vi "Parse Response.vi"(6 "Command String (Hex)":string, 8 "error in (no error)":errorcluster, 10 "Response String (Hex)":string, 11 "Hitronics in":refnum<class "Hitronics.lvclass">) -> (0 "error out":errorcluster, 2 "Response":string, 3 "Hitronics out":refnum<class "Hitronics.lvclass">)   [LabVIEW 2018, in "Hitronics.lvlib" / "Hitronics.lvclass"]
uses:
  Hitronics.lvclass
  Hitronics.lvclass/Hitronics.ctl
panel:
  out "Data":string
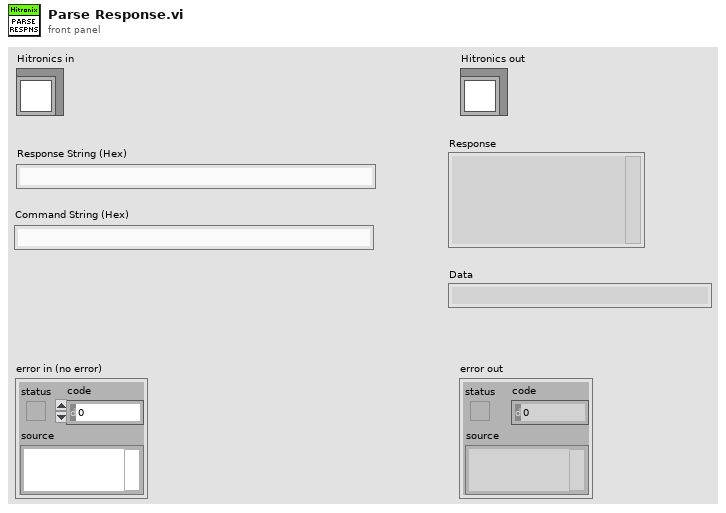
[diagram p1: front panel]
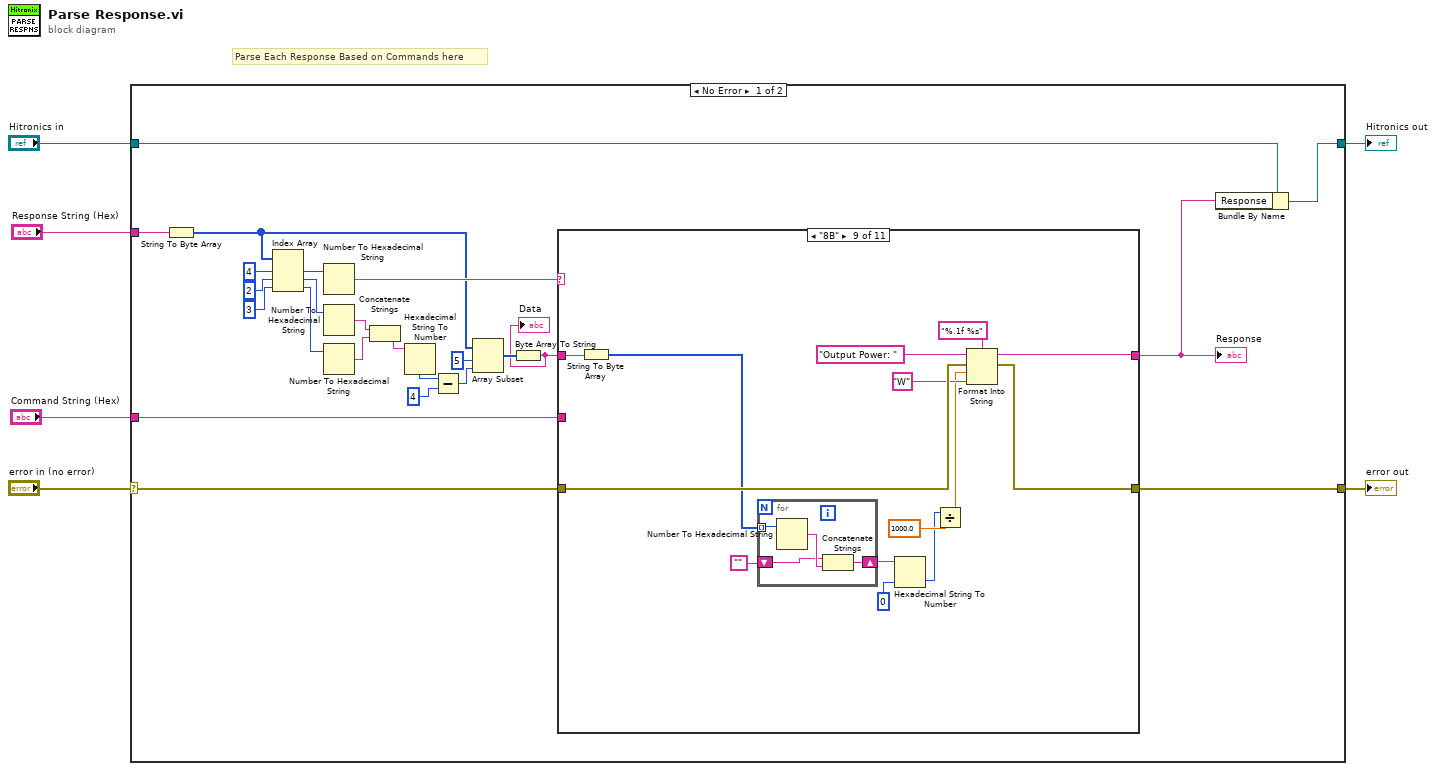
[diagram p0: block diagram]
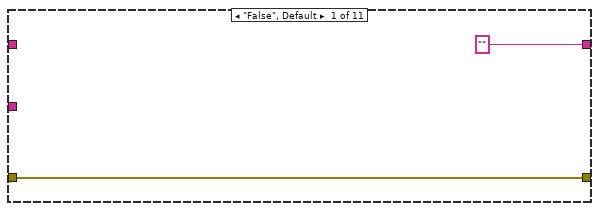
[diagram p2: hidden frame]
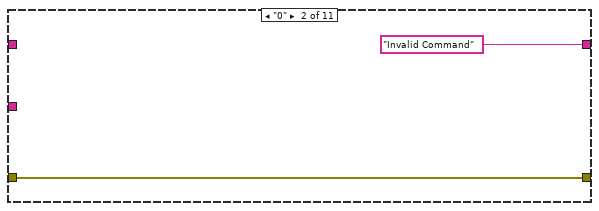
[diagram p3: hidden frame]
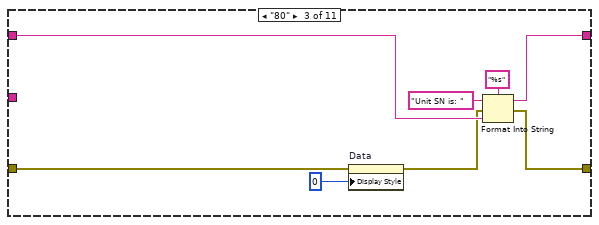
[diagram p4: hidden frame]
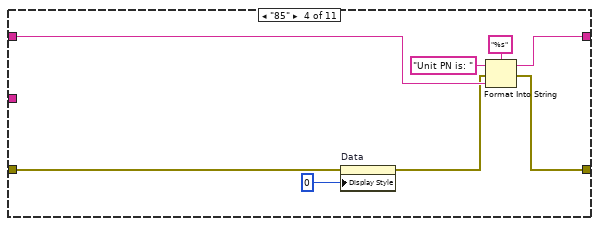
[diagram p5: hidden frame]
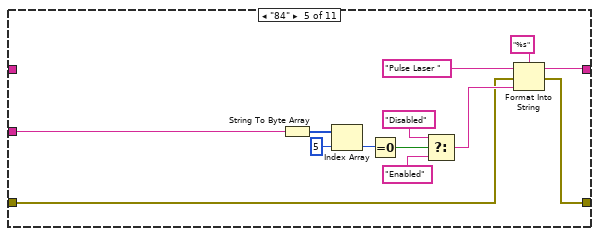
[diagram p6: hidden frame]
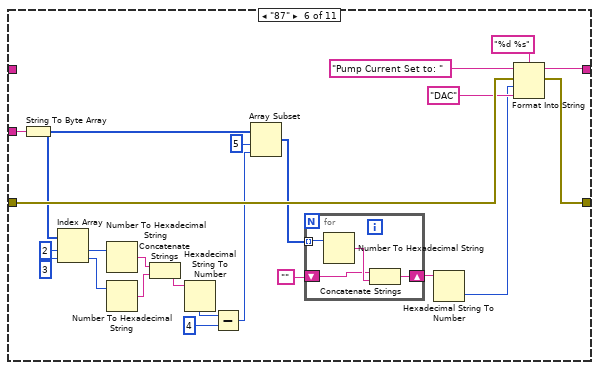
[diagram p7: hidden frame]
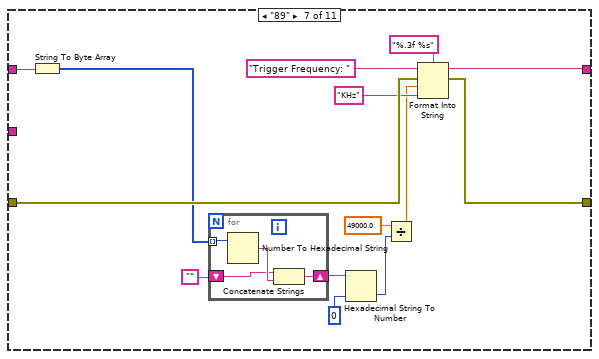
[diagram p8: hidden frame]
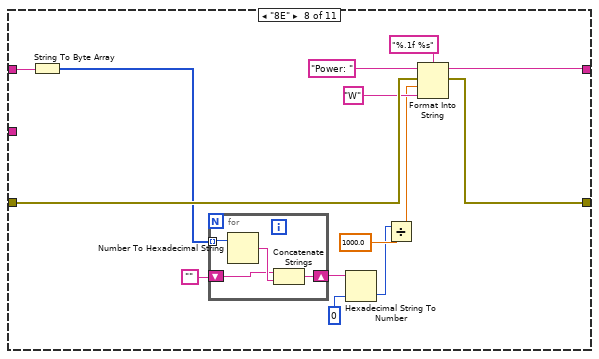
[diagram p9: hidden frame]
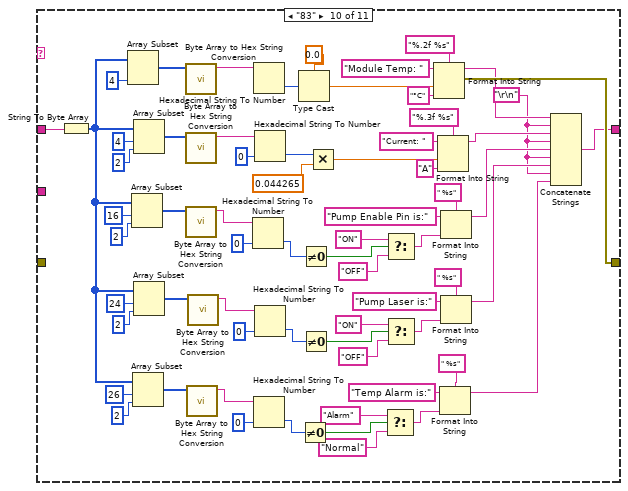
[diagram p10: hidden frame]
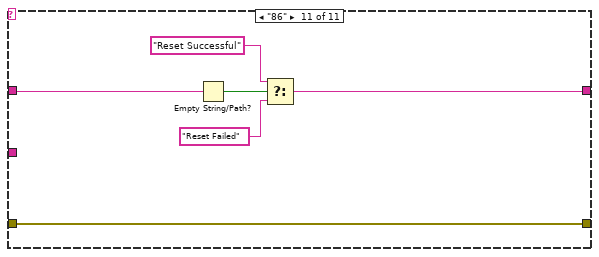
[diagram p11: hidden frame]
diagram:
  # "Parse Each Response Based on Commands here"
  n1 = case shown="No Error" "error in (no error)" {
    selector: "error in (no error)" -> [w12 w218]
    tunnel: [w11 w218] -> w5
    tunnel: [w29 w217] -> w3
    tunnel: "Hitronics in" -> [w30 w217]
    tunnel: "Response String (Hex)" -> [w25 _]
    tunnel: "Command String (Hex)" -> [w8 _]
    frame No Error {
      n2 = String To Byte Array(string=w25) -> (unsigned byte array=w7:u8[])
      n3 = Index Array(array=w7, index #1=4 ("index"), index #2=2 ("index"), index #3=3 ("index")) -> (element #1=w27:u8, element #2=w22:u8, element #3=w21:u8)
      n4 = Number To Hexadecimal String(2:w27) -> (0:w26:string)  [unwired: 1 in]
      n5 = Number To Hexadecimal String(2:w22) -> (0:w20:string)  [unwired: 1 in]
      n6 = Number To Hexadecimal String(2:w21) -> (0:w19:string)  [unwired: 1 in]
      n7 = Concatenate Strings(w20, w19) -> (w18:string)
      n8 = Hexadecimal String To Number(string=w18) -> (number=w17:u32)  [unwired: 2 in, 1 out]
      n9 = Subtract(x=w17, y=u32 4) -> (x-y=w14:u32)
      n10 = Array Subset(array=w7, index=5, length=w14) -> (w13:u8[])
      n11 = Byte Array To String(unsigned byte array=w13) -> (string=w10:string)
      "Data" <- w10
      n12 = case shown="\"8B\"" w26 {
        tunnel: ["" "Invalid Command" w37 w45 w53 w84 w102 w120 w138 w189 w212] -> w9
        tunnel: w10 -> [_ _ w39 w46 _ _ w92 w110 w128 w205 w216]
        tunnel: w12 -> [w31 w33 w41 w49 w52 w83 w101 w119 w137 _ w211]
        tunnel: [w31 w33 w35 w43 w51 w82 w100 w118 w136 w208 w211] -> w11
        tunnel: w8 -> [_ _ _ _ w63 w81 _ _ _ _ _]
        frame "False", Default {
        }
        frame "0" {
        }
        frame "80" {
          n13 = property on="Data" class="Str"(error in=w41, "Display Style"=u32 0) -> (error out=w36:errorcluster)  [unwired: 1 in, 1 out]
          n14 = Format Into String(format string="%s", initial string="Unit SN is: ", error in=w36, w39) -> (resulting string=w37:string, error out=w35:errorcluster)
        }
        frame "85" {
          n15 = property on="Data" class="Str"(error in=w49, "Display Style"=u32 0) -> (error out=w44:errorcluster)  [unwired: 1 in, 1 out]
          n16 = Format Into String(format string="%s", initial string="Unit PN is: ", error in=w44, w46) -> (resulting string=w45:string, error out=w43:errorcluster)
        }
        frame "84" {
          n17 = String To Byte Array(string=w63) -> (unsigned byte array=w62:u8[])
          n18 = Index Array(array=w62, index=5) -> (element=w60:u8)
          n19 = Equal To 0?(x=w60) -> (x = 0?=w59:bool)
          n20 = Select(t="Disabled", s=w59, f="Enabled") -> (s? t:f=w54:string)
          n21 = Format Into String(format string="%s", initial string="Pulse Laser ", error in=w52, w54) -> (resulting string=w53:string, error out=w51:errorcluster)
        }
        frame "87" {
          n22 = String To Byte Array(string=w81) -> (unsigned byte array=w78:u8[])
          n23 = Index Array(array=w78, index #1=2 ("index"), index #2=3 ("index")) -> (element #1=w70:u8, element #2=w69:u8)
          n24 = Number To Hexadecimal String(2:w70) -> (0:w71:string)  [unwired: 1 in]
          n25 = Number To Hexadecimal String(2:w69) -> (0:w72:string)  [unwired: 1 in]
          n26 = Concatenate Strings(w71, w72) -> (w73:string)
          n27 = Hexadecimal String To Number(string=w73) -> (number=w74:u32)  [unwired: 2 in, 1 out]
          n28 = Subtract(x=w74, y=u32 4) -> (x-y=w68:u32)
          n29 = Array Subset(array=w78, index=5, length=w68) -> (w67:u8[])
          n30 = for {
            tunnel: w67 -> [w90] mode=indexing
            shift-right: [w87] -> w66
            shift-left: "" -> [w88]
            n31 = Number To Hexadecimal String(2:w90) -> (0:w89:string)  [unwired: 1 in]
            n32 = Concatenate Strings(w88, w89) -> (w87:string)
          }
          n33 = Hexadecimal String To Number(string=w66) -> (number=w65:u32)  [unwired: 2 in, 1 out]
          n34 = Format Into String(format string="%d %s", initial string="Pump Current Set to: ", error in=w83, w65, "DAC") -> (resulting string=w84:string, error out=w82:errorcluster)
        }
        frame "89" {
          n35 = String To Byte Array(string=w92) -> (unsigned byte array=w91:u8[])
          n36 = for {
            tunnel: w91 -> [w108] mode=indexing
            shift-right: [w105] -> w98
            shift-left: "" -> [w106]
            n37 = Number To Hexadecimal String(2:w108) -> (0:w107:string)  [unwired: 1 in]
            n38 = Concatenate Strings(w106, w107) -> (w105:string)
          }
          n39 = Hexadecimal String To Number(string=w98, default (0uL)=i16 0) -> (number=w95:i16)  [unwired: 1 in, 1 out]
          n40 = Divide(x=49000.0, y=w95) -> (x/y=w94:dbl)
          n41 = Format Into String(format string="%.3f %s", initial string="Trigger Frequency: ", error in=w101, w94, "KHz") -> (resulting string=w102:string, error out=w100:errorcluster)
        }
        frame "8E" {
          n42 = String To Byte Array(string=w110) -> (unsigned byte array=w109:u8[])
          n43 = for {
            tunnel: w109 -> [w126] mode=indexing
            shift-right: [w123] -> w116
            shift-left: "" -> [w124]
            n44 = Number To Hexadecimal String(2:w126) -> (0:w125:string)  [unwired: 1 in]
            n45 = Concatenate Strings(w124, w125) -> (w123:string)
          }
          n46 = Hexadecimal String To Number(string=w116, default (0uL)=i16 0) -> (number=w113:i16)  [unwired: 1 in, 1 out]
          n47 = Divide(x=w113, y=1000.0) -> (x/y=w112:dbl)
          n48 = Format Into String(format string="%.1f %s", initial string="Power: ", error in=w119, w112, "W") -> (resulting string=w120:string, error out=w118:errorcluster)
        }
        frame "8B" {
          n49 = String To Byte Array(string=w128) -> (unsigned byte array=w127:u8[])
          n50 = for {
            tunnel: w127 -> [w144] mode=indexing
            shift-right: [w141] -> w134
            shift-left: "" -> [w142]
            n51 = Number To Hexadecimal String(2:w144) -> (0:w143:string)  [unwired: 1 in]
            n52 = Concatenate Strings(w142, w143) -> (w141:string)
          }
          n53 = Hexadecimal String To Number(string=w134, default (0uL)=i16 0) -> (number=w131:i16)  [unwired: 1 in, 1 out]
          n54 = Divide(x=w131, y=1000.0) -> (x/y=w130:dbl)
          n55 = Format Into String(format string="%.1f %s", initial string="Output Power: ", error in=w137, w130, "W") -> (resulting string=w138:string, error out=w136:errorcluster)
        }
        frame "83" {
          w145 = "\r\n"
          n56 = String To Byte Array(string=w205) -> (unsigned byte array=w148:u8[])
          n57 = Array Subset(array=w148, length=4) -> (w203:u8[])  [unwired: 1 in]
          n58 = Array Subset(array=w148, index=16, length=2) -> (w183:u8[])
          n59 = Array Subset(array=w148, index=26, length=2) -> (w151:u8[])
          n60 = Array Subset(array=w148, index=4, length=2) -> (w200:u8[])
          n61 = Array Subset(array=w148, index=24, length=2) -> (w170:u8[])
          n62 = call "Byte Array to Hex String Conversion.vi"("Array"=w203) -> ("String"=w206:string)  [unwired: 9 in, 1 out]
          n63 = call "Byte Array to Hex String Conversion.vi"("Array"=w200) -> ("String"=w198:string)  [unwired: 9 in, 1 out]
          n64 = call "Byte Array to Hex String Conversion.vi"("Array"=w183) -> ("String"=w178:string)  [unwired: 9 in, 1 out]
          n65 = call "Byte Array to Hex String Conversion.vi"("Array"=w151) -> ("String"=w150:string)  [unwired: 9 in, 1 out]
          n66 = call "Byte Array to Hex String Conversion.vi"("Array"=w170) -> ("String"=w171:string)  [unwired: 9 in, 1 out]
          n67 = Hexadecimal String To Number(string=w178, default (0uL)=i16 0 ("default (0 U32)")) -> (number=w176:i16)  [unwired: 1 in, 1 out]
          n68 = Hexadecimal String To Number(string=w206) -> (number=w187:u32)  [unwired: 2 in, 1 out]
          n69 = Hexadecimal String To Number(string=w150, default (0uL)=i16 0 ("default (0 U32)")) -> (number=w159:i16)  [unwired: 1 in, 1 out]
          n70 = Hexadecimal String To Number(string=w198, default (0uL)=u16 0 ("Numeric")) -> (number=w197:u16)  [unwired: 1 in, 1 out]
          n71 = Hexadecimal String To Number(string=w171, default (0uL)=i16 0 ("default (0 U32)")) -> (number=w161:i16)  [unwired: 1 in, 1 out]
          n72 = Type Cast(type=sgl 0.0 ("Numeric"), x=w187) -> (*(type *) &x=w186:sgl)
          n73 = Not Equal To 0?(x=w159) -> (x != 0?=w155:bool)
          n74 = Not Equal To 0?(x=w176) -> (x != 0?=w175:bool)
          n75 = Not Equal To 0?(x=w161) -> (x != 0?=w166:bool)
          n76 = Multiply(x=w197, y=0.044265) -> (x*y=w192:dbl)
          n77 = Select(t="Alarm", s=w155, f="Normal") -> (s? t:f=w154:string)
          n78 = Select(t="ON", s=w175, f="OFF") -> (s? t:f=w174:string)
          n79 = Select(t="ON", s=w166, f="OFF") -> (s? t:f=w167:string)
          n80 = Format Into String(format string="%.2f %s", initial string="Module Temp: ", w186, "°C") -> (resulting string=w191:string, error out=w208:errorcluster)  [unwired: 1 in]
          n81 = Format Into String(format string="%.3f %s", initial string="Current: ", w192, "A") -> (resulting string=w190:string)  [unwired: 1 in, 1 out]
          n82 = Format Into String(format string=" %s", initial string="Temp Alarm is:", w154) -> (resulting string=w146:string)  [unwired: 1 in, 1 out]
          n83 = Format Into String(format string=" %s", initial string="Pump Enable Pin is:", w174) -> (resulting string=w173:string)  [unwired: 1 in, 1 out]
          n84 = Format Into String(format string=" %s", initial string="Pump Laser is:", w167) -> (resulting string=w160:string)  [unwired: 1 in, 1 out]
          n85 = Concatenate Strings(w191, w145, w190, w145, w173, w145, w160, w145, w146) -> (w189:string)
        }
        frame "86" {
          n86 = Empty String/Path?(string/path=w216) -> (empty?=w215:bool)
          n87 = Select(t="Reset Successful", s=w215, f="Reset Failed") -> (s? t:f=w212:string)
        }
      }
      "Response" <- w9
      n88 = Bundle By Name(cluster=w30, "Response"=w9) -> (w29:refnum<class "Hitronics.lvclass">)
    }
    frame Error {
    }
  }
  "error out" <- w5
  "Hitronics out" <- w3
